vi "_getParam.vi"(5 "default value":string, 6 "param name":string="filename", 7 "xml string":string) -> (3 "param value":string)   [LabVIEW 2020]
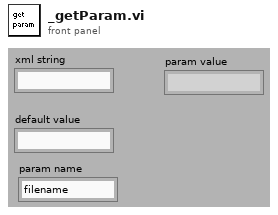
[diagram p1: front panel]
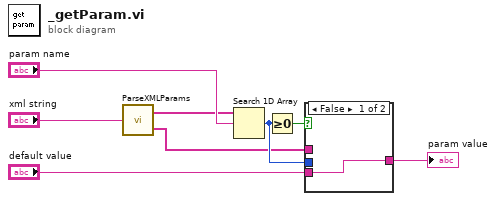
[diagram p0: block diagram]
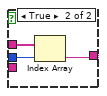
[diagram p2: hidden frame]
diagram:
  n1 = call <vilib>:"ParseXMLParams.vi"("Parameter String"="xml string") -> ("Names"=w2:string[], "Values"=w5:string[])
  n2 = Search 1D Array(1D array=w2, element="param name") -> (index of element=w6:i32)  [unwired: 1 in]
  n3 = Greater Or Equal To 0?(x=w6) -> (x >= 0?=w4:bool)
  n4 = case shown="False" w4 {
    tunnel: w5 -> [_ w12]
    tunnel: w6 -> [_ w11]
    tunnel: [w9 w10] -> w8
    tunnel: "default value" -> [w9 _]
    frame False {
    }
    frame True {
      n5 = Index Array(array=w12, index=w11) -> (element=w10:string)
    }
  }
  "param value" <- w8
